vi "UI_Set_startup_controls_state_(01).vi"(3 "error in (no error)":errorcluster, 4 "Settings cluster in":T1={"Defaults"={"Default User"=0.0, "VISA Resource Name "=""}, "Recording and saving"={"Researcher name"="", "Name prefix"="", "Data filtering"=0, "Stop at"=0.0, "\"Stop at\" enabled"=FALSE}, "Geometry"={"Cage diameter, mm"=0, "Starting angle MIDFIELD"=0, "Starting angle BORDER"=0, "Radius, mm CENTER"=0, "Radius, mm MIDFIELD"=0, "N segments MIDFIELD"=0, "N segments BORDER"=0, "R-gap, mm"=0.0, "Bridge swap"=FALSE, "Bridge H. offset"=0.0, "Bridge V. offset"=0.0, "Twisted neck"=FALSE}, "IO parameters"={"SYNC configuration"=0, "IO 1 configuration"=0, "IO 2 configuration"=0, "IO 3 configuration"=0, "IO 4 configuration"=0, "Activate ext. RS-232"=0, "IO inversion config."=0}, "Stimulus presets array"=[{"Event type"=0, "Dur., s"=0.0, "Stim., s"=0.0, "TTL out N"=1, "Set/Clear"=FALSE, "Stim. has been set"=FALSE}, {"Event type"=0, "Dur., s"=0.0, "Stim., s"=0.0, "TTL out N"=1, "Set/Clear"=FALSE, "Stim. has been set"=FALSE}, {"Event type"=0, "Dur., s"=0.0, "Stim., s"=0.0, "TTL out N"=1, "Set/Clear"=FALSE, "Stim. has been set"=FALSE}, {"Event type"=0, "Dur., s"=0.0, "Stim., s"=0.0, "TTL out N"=1, "Set/Clear"=FALSE, "Stim. has been set"=FALSE}, {"Event type"=0, "Dur., s"=0.0, "Stim., s"=0.0, "TTL out N"=1, "Set/Clear"=FALSE, "Stim. has been set"=FALSE}, {"Event type"=0, "Dur., s"=0.0, "Stim., s"=0.0, "TTL out N"=1, "Set/Clear"=FALSE, "Stim. has been set"=FALSE}, {"Event type"=0, "Dur., s"=0.0, "Stim., s"=0.0, "TTL out N"=1, "Set/Clear"=FALSE, "Stim. has been set"=FALSE}, {"Event type"=0, "Dur., s"=0.0, "Stim., s"=0.0, "TTL out N"=1, "Set/Clear"=FALSE, "Stim. has been set"=FALSE}, {"Event type"=0, "Dur., s"=0.0, "Stim., s"=0.0, "TTL out N"=1, "Set/Clear"=FALSE, "Stim. has been set"=FALSE}, {"Event type"=0, "Dur., s"=0.0, "Stim., s"=0.0, "TTL out N"=1, "Set/Clear"=FALSE, "Stim. has been set"=FALSE}, {"Event type"=0, "Dur., s"=0.0, "Stim., s"=0.0, "TTL out N"=1, "Set/Clear"=FALSE, "Stim. has been set"=FALSE}, {"Event type"=0, "Dur., s"=0.0, "Stim., s"=0.0, "TTL out N"=1, "Set/Clear"=FALSE, "Stim. has been set"=FALSE}, {"Event type"=0, "Dur., s"=0.0, "Stim., s"=0.0, "TTL out N"=1, "Set/Clear"=FALSE, "Stim. has been set"=FALSE}, {"Event type"=0, "Dur., s"=0.0, "Stim., s"=0.0, "TTL out N"=1, "Set/Clear"=FALSE, "Stim. has been set"=FALSE}], "Settings loaded OK"=FALSE} {"Stimulus presets array"."Event type" items=["Stay for N seconds"]; "Stimulus presets array"."TTL out N" items=["1"=1, "2"=2, "1+2"=3]; "Geometry"."Cage diameter, mm" scale=0.0..340.0}, 5 "All references in":T5) -> (0 "error out":errorcluster, 1 "Settings cluster out":T1={"Defaults"={"Default User"=0.0, "VISA Resource Name "=""}, "Recording and saving"={"Researcher name"="", "Name prefix"="", "Data filtering"=0, "Stop at"=0.0, "\"Stop at\" enabled"=FALSE}, "Geometry"={"Cage diameter, mm"=0, "Starting angle MIDFIELD"=0, "Starting angle BORDER"=0, "Radius, mm CENTER"=0, "Radius, mm MIDFIELD"=0, "N segments MIDFIELD"=0, "N segments BORDER"=0, "R-gap, mm"=0.0, "Bridge swap"=FALSE, "Bridge H. offset"=0.0, "Bridge V. offset"=0.0, "Twisted neck"=FALSE}, "IO parameters"={"SYNC configuration"=0, "IO 1 configuration"=0, "IO 2 configuration"=0, "IO 3 configuration"=0, "IO 4 configuration"=0, "Activate ext. RS-232"=0, "IO inversion config."=0}, "Stimulus presets array"=[{"Event type"=0, "Dur., s"=0.0, "Stim., s"=0.0, "TTL out N"=1, "Set/Clear"=FALSE, "Stim. has been set"=FALSE}, {"Event type"=0, "Dur., s"=0.0, "Stim., s"=0.0, "TTL out N"=1, "Set/Clear"=FALSE, "Stim. has been set"=FALSE}, {"Event type"=0, "Dur., s"=0.0, "Stim., s"=0.0, "TTL out N"=1, "Set/Clear"=FALSE, "Stim. has been set"=FALSE}, {"Event type"=0, "Dur., s"=0.0, "Stim., s"=0.0, "TTL out N"=1, "Set/Clear"=FALSE, "Stim. has been set"=FALSE}, {"Event type"=0, "Dur., s"=0.0, "Stim., s"=0.0, "TTL out N"=1, "Set/Clear"=FALSE, "Stim. has been set"=FALSE}, {"Event type"=0, "Dur., s"=0.0, "Stim., s"=0.0, "TTL out N"=1, "Set/Clear"=FALSE, "Stim. has been set"=FALSE}, {"Event type"=0, "Dur., s"=0.0, "Stim., s"=0.0, "TTL out N"=1, "Set/Clear"=FALSE, "Stim. has been set"=FALSE}, {"Event type"=0, "Dur., s"=0.0, "Stim., s"=0.0, "TTL out N"=1, "Set/Clear"=FALSE, "Stim. has been set"=FALSE}, {"Event type"=0, "Dur., s"=0.0, "Stim., s"=0.0, "TTL out N"=1, "Set/Clear"=FALSE, "Stim. has been set"=FALSE}, {"Event type"=0, "Dur., s"=0.0, "Stim., s"=0.0, "TTL out N"=1, "Set/Clear"=FALSE, "Stim. has been set"=FALSE}, {"Event type"=0, "Dur., s"=0.0, "Stim., s"=0.0, "TTL out N"=1, "Set/Clear"=FALSE, "Stim. has been set"=FALSE}, {"Event type"=0, "Dur., s"=0.0, "Stim., s"=0.0, "TTL out N"=1, "Set/Clear"=FALSE, "Stim. has been set"=FALSE}, {"Event type"=0, "Dur., s"=0.0, "Stim., s"=0.0, "TTL out N"=1, "Set/Clear"=FALSE, "Stim. has been set"=FALSE}, {"Event type"=0, "Dur., s"=0.0, "Stim., s"=0.0, "TTL out N"=1, "Set/Clear"=FALSE, "Stim. has been set"=FALSE}], "Settings loaded OK"=FALSE} {"Stimulus presets array"."Event type" items=["Stay for N seconds"]; "Stimulus presets array"."TTL out N" items=["1"=1, "2"=2, "1+2"=3]; "Geometry"."Cage diameter, mm" scale=0.0..340.0}, 2 "All references out":T5)   [LabVIEW 2018]
uses:
  Controls/CTL_All_References.ctl
  Controls/CTL_Controls_References.ctl
  Controls/CTL_Indicators_References.ctl
  Controls/CTL_Panes_and_VIs_References.ctl
  Controls/CTL_Histogram_Properties.ctl
  <vilib>/Utility/miscctls.llb/LVRangeTypeDef.ctl
  Controls/CTL_Settings_cluster.ctl
  Controls/CTL_Single_stimulus_setting.ctl
  <vilib>/Utility/error.llb/Error Cluster From Error Code.vi
  <vilib>/ErrorRing/Error Ring.xnode
panel:
  out "Erroneous ref name":string
  in  "Histogram initialization cluster":T3={"X Scale.Range"={"Minimum"=0.0, "Maximum"=13.0, "Increment"=1.0, "Minor Increment"=1.0, "Start"=0.0}, "Caption.Text"="Zone preference (normalized)", "X Scale.Offset and Multiplier:Multiplier"=1.0, "X Scale.Offset and Multiplier:Offset"=0.0, "X Scale.Scale Fit"=2, "X Scale.Display Format:Precision"=0, "Y Scale.Mapping Mode"=0, "Zones preference empty initialized array"=[0, 0, 0, 0, 0, 0, 0, 0, 0, 0, 0, 0, 0, 0], "Plot.Fill/Point Color"=15790320}
  out "Panes references":T8
  out "Controls references params":string[][](array[string])
  out "Indicators references params":string[][](array[string])
  out "Indicators references":T7
  out "Controls references":T6
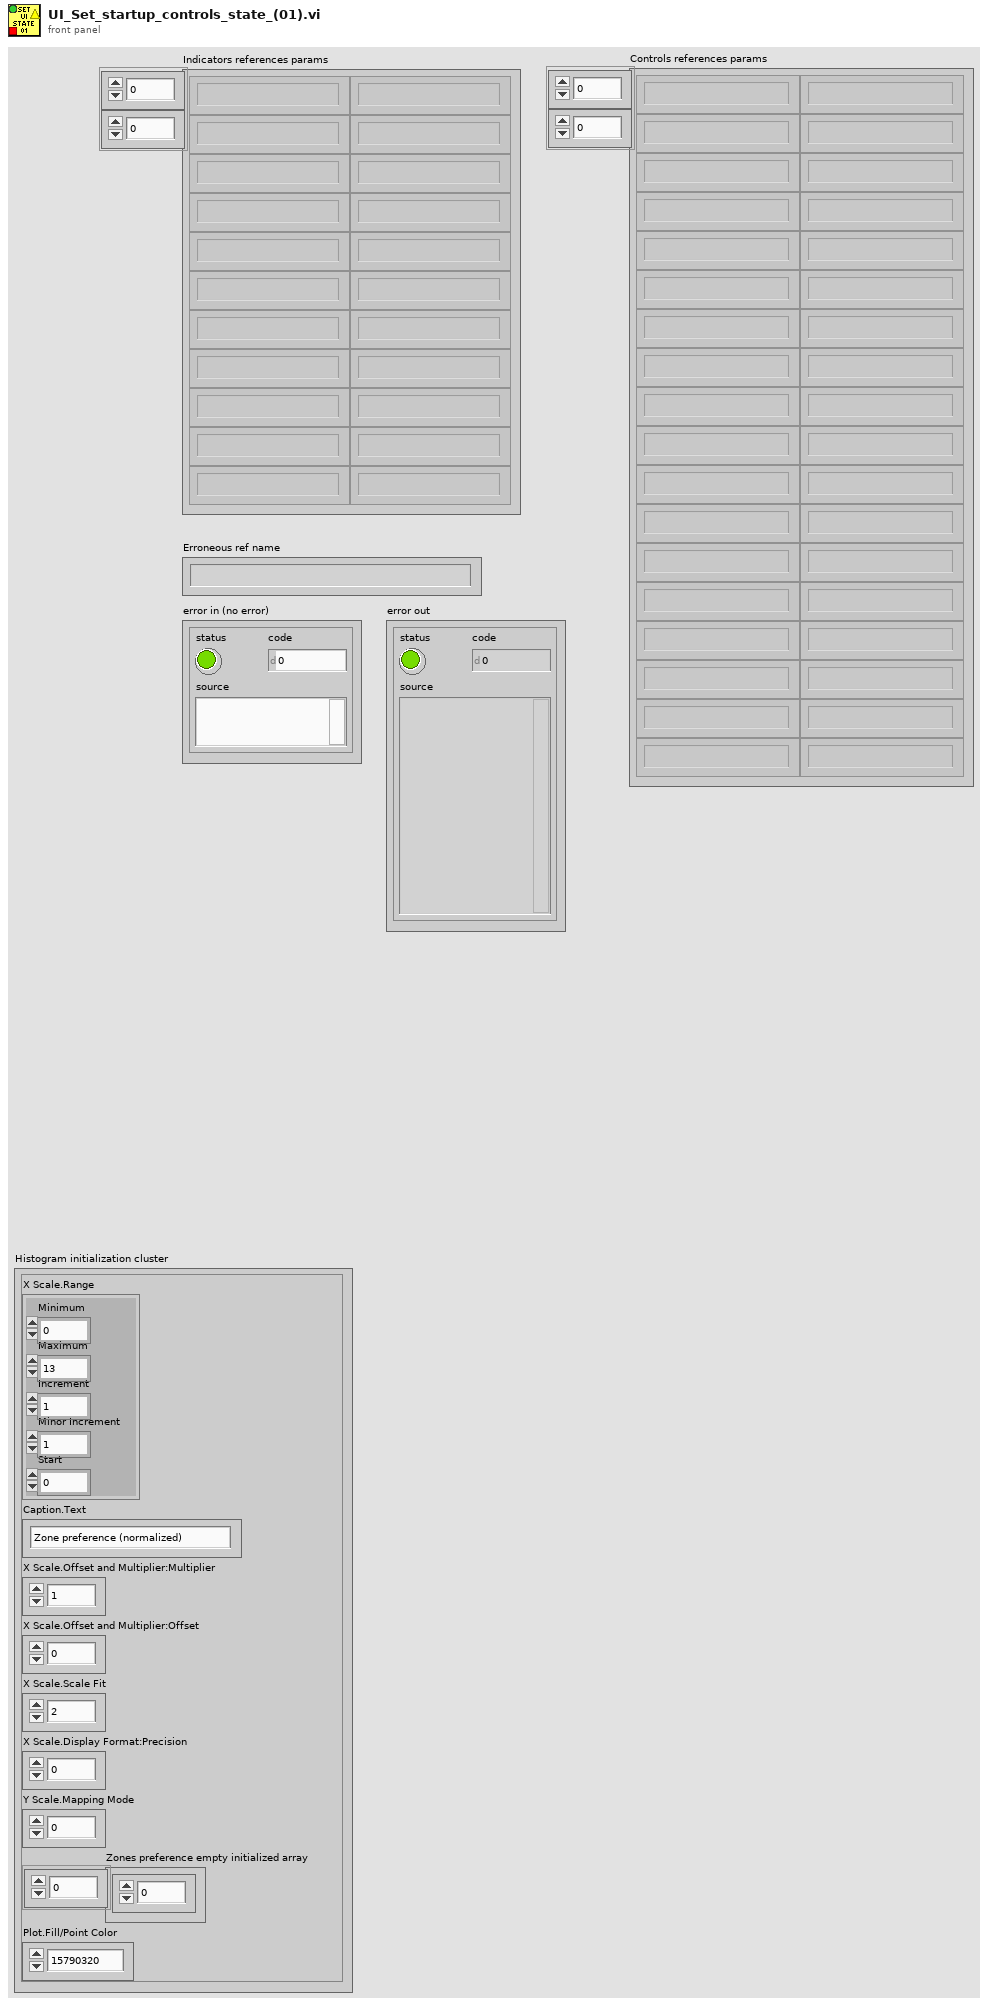
[diagram p1: front panel]
types:
  T1 = typedef "CTL_Settings_cluster.ctl" = cluster{"Defaults":cluster{"Default User":dbl, "VISA Resource Name ":string}, "Recording and saving":cluster{"Researcher name":string, "Name prefix":string, "Data filtering":u16, "Stop at":dbl, "\"Stop at\" enabled":bool}, "Geometry":cluster{"Cage diameter, mm":u16, "Starting angle MIDFIELD":i16, "Starting angle BORDER":i16, "Radius, mm CENTER":u16, "Radius, mm MIDFIELD":u16, "N segments MIDFIELD":u8, "N segments BORDER":u8, "R-gap, mm":sgl, "Bridge swap":bool, "Bridge H. offset":sgl, "Bridge V. offset":sgl, "Twisted neck":bool}, "IO parameters":cluster{"SYNC configuration":u16, "IO 1 configuration":u16, "IO 2 configuration":u16, "IO 3 configuration":u16, "IO 4 configuration":u16, "Activate ext. RS-232":u16, "IO inversion config.":u16}, "Stimulus presets array":T2[], "Settings loaded OK":bool}
  T2 = typedef "CTL_Single_stimulus_setting.ctl" = cluster{"Event type":u16, "Dur., s":sgl, "Stim., s":sgl, "TTL out N":u16, "Set/Clear":bool, "Stim. has been set":bool}
  T3 = typedef "CTL_Histogram_Properties.ctl" = cluster{"X Scale.Range":T4, "Caption.Text":string, "X Scale.Offset and Multiplier:Multiplier":dbl, "X Scale.Offset and Multiplier:Offset":dbl, "X Scale.Scale Fit":u8, "X Scale.Display Format:Precision":u8, "Y Scale.Mapping Mode":u8, "Zones preference empty initialized array":i32[], "Plot.Fill/Point Color":u32}
  T4 = typedef "LVRangeTypeDef.ctl" = cluster{"Minimum":dbl, "Maximum":dbl, "Increment":dbl, "Minor Increment":dbl, "Start":dbl}
  T5 = typedef "CTL_All_References.ctl" = cluster{"Controls references":T6, "Indicators references":T7, "Panes references":T8}
  T6 = typedef "CTL_Controls_References.ctl" = cluster{"Check HW connection":refnum<vi>, "Start Tracking button":refnum<vi>, "Reset zones":refnum<vi>, "Reset stimuli":refnum<vi>, "Record/Stop":refnum<vi>, "Reset barplot":refnum<vi>, "Multiplyer of chart RX":refnum<vi>, "Show zones":refnum<vi>, "Show magnets":refnum<vi>, "Show heatmap":refnum<vi>, "Show full track":refnum<vi>, "Open File":refnum<vi>, "Play/Pause":refnum<vi>, "Trace, s":refnum<vi>, "Playback speed":refnum<vi>, "Timeline":refnum<vi>, "By Zone stim. setup":refnum<vi>}
  T7 = typedef "CTL_Indicators_References.ctl" = cluster{"HW info":refnum<vi>, "Port":refnum<vi>, "Ready":refnum<vi>, "IO status indicator":refnum<vi>, "Current Time":refnum<vi>, "Record timestamp":refnum<vi>, "Mouse speed":refnum<vi>, "Mouse speed, mm/s":refnum<vi>, "Running, perc. of time":refnum<vi>, "Histograms":refnum<vi>}
  T8 = typedef "CTL_Panes_and_VIs_References.ctl" = cluster{"Pane":refnum<vi>, "This VI":refnum<vi>}
  T9 = cluster{"SYNC configuration":u16, "IO 1 configuration":u16, "IO 2 configuration":u16, "IO 3 configuration":u16, "IO 4 configuration":u16, "Activate ext. RS-232":u16, "IO inversion config.":u16}
  T10 = enum8{"Enabled", "Disabled", "Disabled and Grayed Out"}
  T11 = typedef "CTL_IO_parameters_indicator.ctl" = cluster{"IO1":bool, "IO2":bool, "IO3":bool, "IO4":bool, "Z1":bool, "Z2":bool, "Z3":bool, "Z4":bool, "St1":bool, "St2":bool, "St3":bool, "St4":bool, "Syn1":bool, "Syn2":bool, "RS-232 ext. activated":bool}
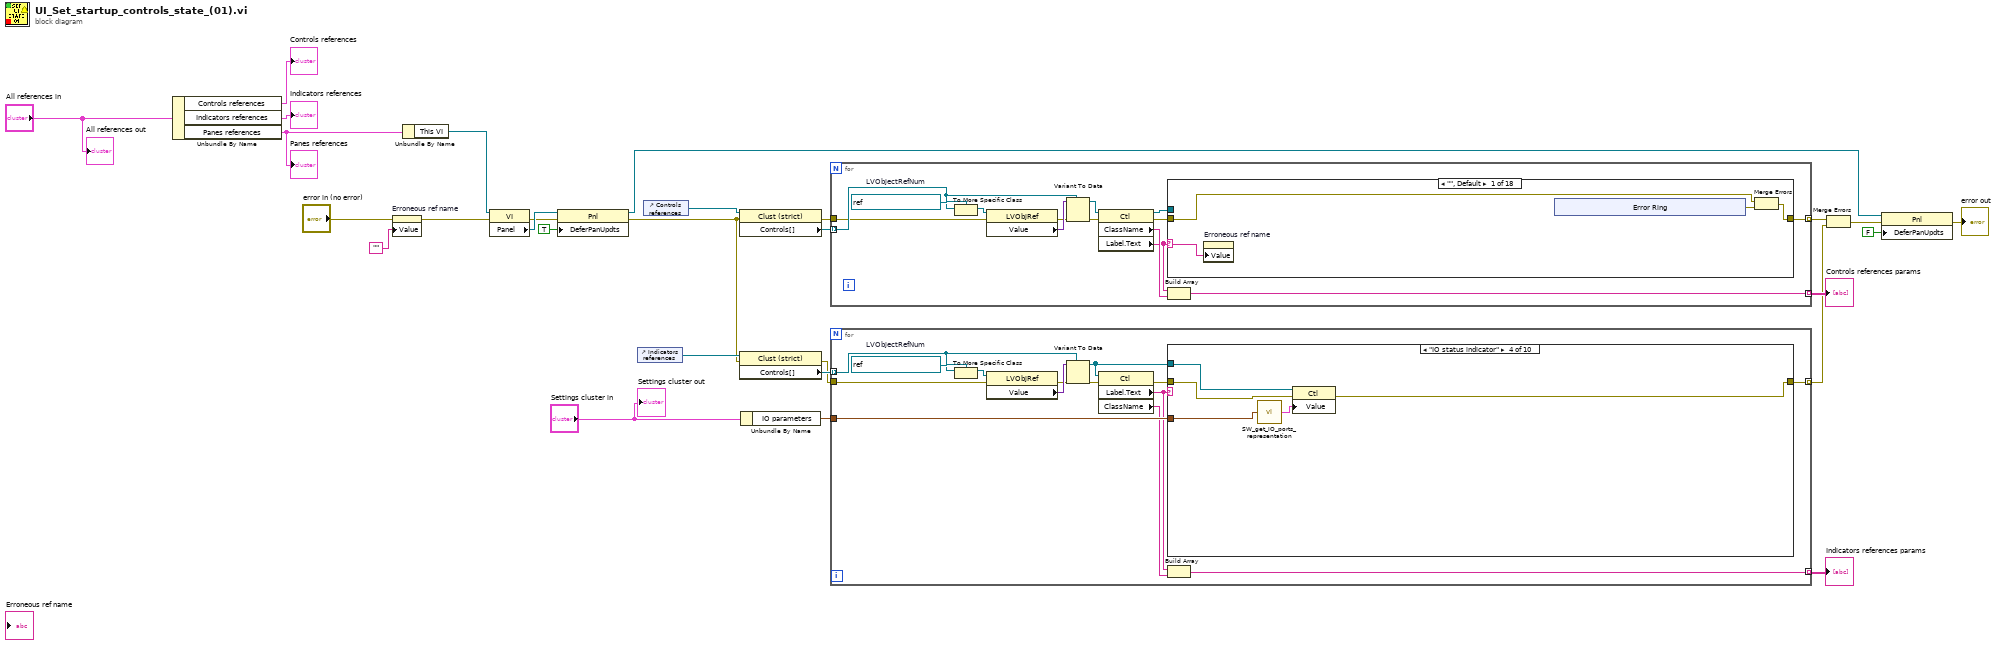
[diagram p0: block diagram]
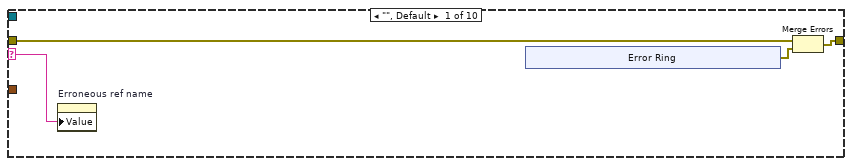
[diagram p2: hidden frame]
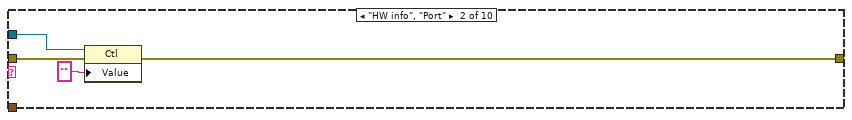
[diagram p3: hidden frame]
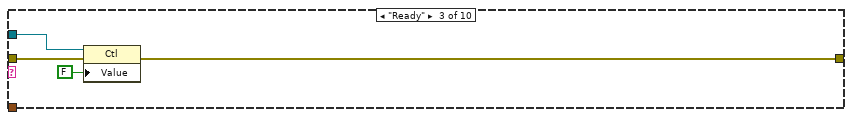
[diagram p4: hidden frame]
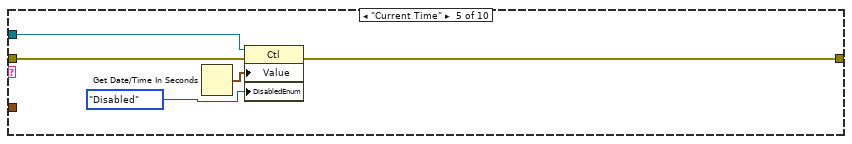
[diagram p5: hidden frame]
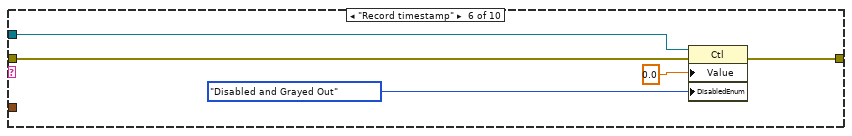
[diagram p6: hidden frame]
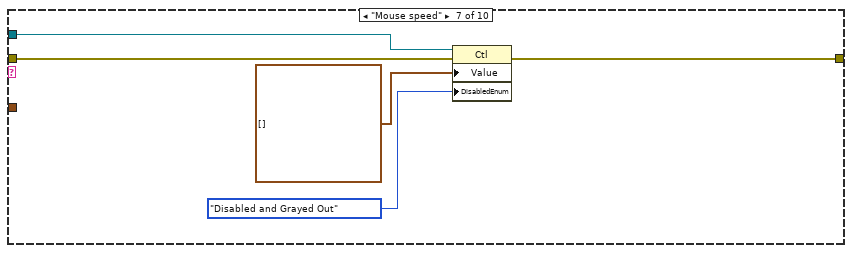
[diagram p7: hidden frame]
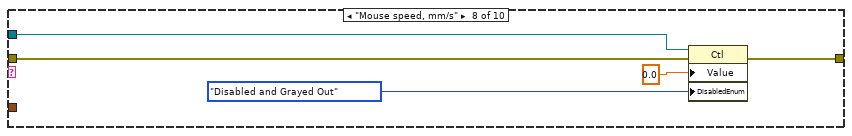
[diagram p8: hidden frame]
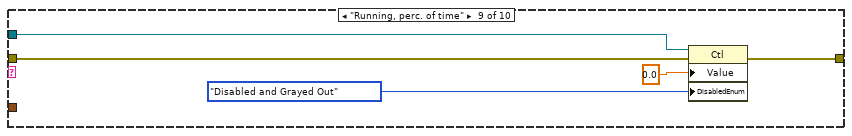
[diagram p9: hidden frame]
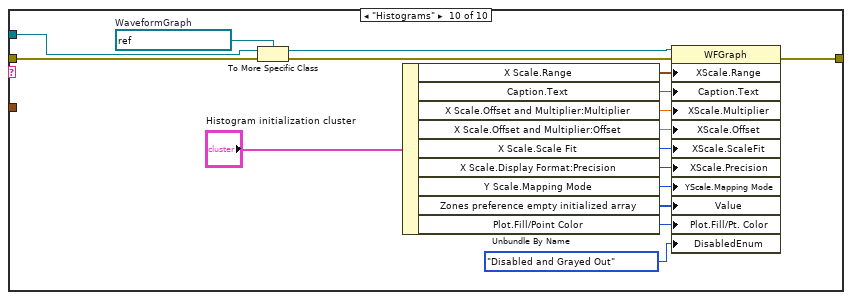
[diagram p10: hidden frame]
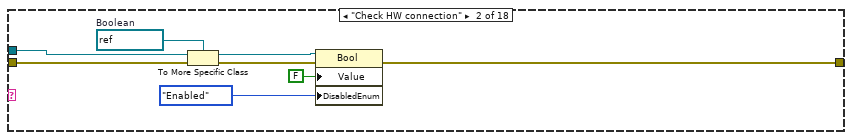
[diagram p11: hidden frame]
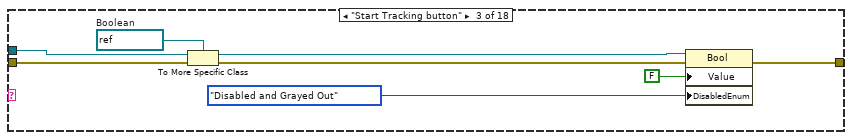
[diagram p12: hidden frame]
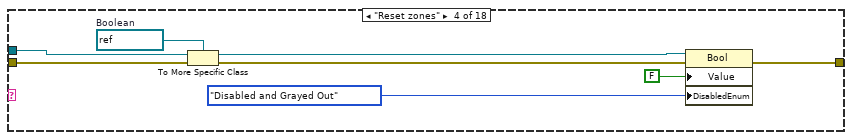
[diagram p13: hidden frame]
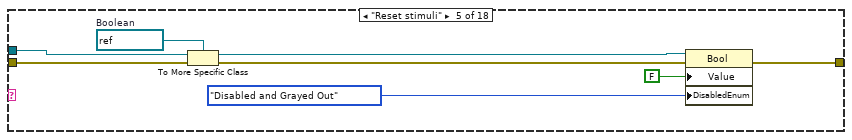
[diagram p14: hidden frame]
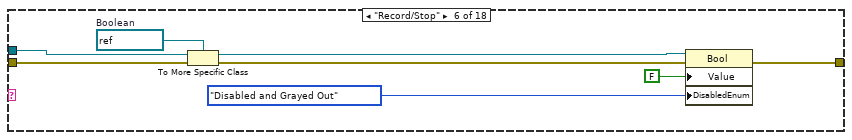
[diagram p15: hidden frame]
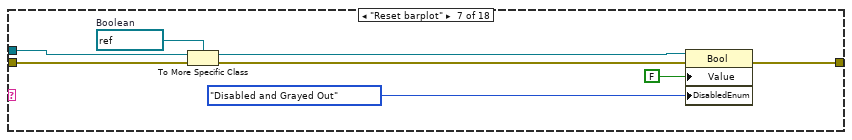
[diagram p16: hidden frame]
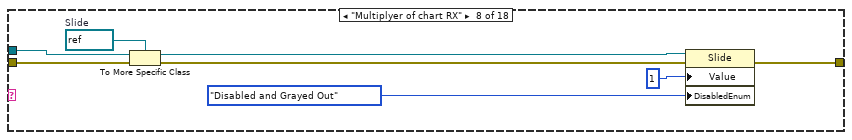
[diagram p17: hidden frame]
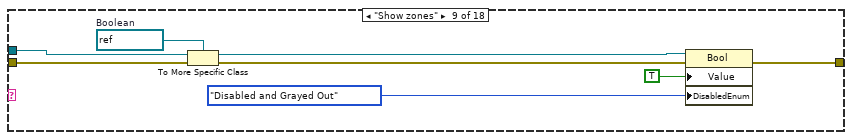
[diagram p18: hidden frame]
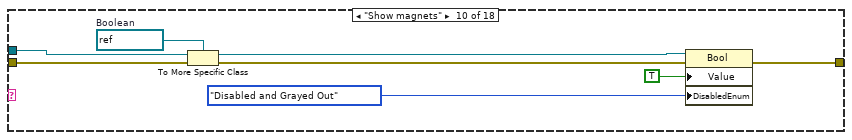
[diagram p19: hidden frame]
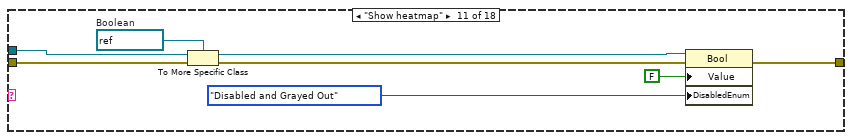
[diagram p20: hidden frame]
diagram:
  n1 = Unbundle By Name("All references in") -> ("Controls references"=→"Controls references":T6, "Indicators references"=→"Indicators references":T7, "Panes references"=w19:T8)
  "Panes references" <- w19
  n2 = property on="Erroneous ref name" class="Str"(error in="error in (no error)", "Value"="") -> (error out=w3:errorcluster)  [unwired: 1 in, 1 out]
  n3 = Unbundle By Name(w19) -> ("This VI"=w16:refnum<vi>)
  n4 = property class="VI"(reference=w16, error in=w3) -> (error out=w8:errorcluster, "Panel"=w18:refnum<vi>)  [unwired: 1 out]
  n5 = property class="Pnl"(reference=w18, error in=w8, "DeferPanUpdts"=TRUE ("Defer Panel Updates")) -> (reference out=w9:refnum<vi>, error out=w15:errorcluster)
  n6 = control-ref of="Indicators references"() -> (w22:refnum<vi>)
  n7 = control-ref of="Controls references"() -> (w24:refnum<vi>)
  n8 = property class="Clust (strict)"(reference=w24, error in=w15) -> (error out=w14:errorcluster, "Controls[]"=w25:refnum<vi>[])  [unwired: 1 out]
  n9 = property class="Clust (strict)"(reference=w22, error in=w15) -> (error out=w13:errorcluster, "Controls[]"=w23:refnum<vi>[])  [unwired: 1 out]
  n10 = Unbundle By Name("Settings cluster in") -> ("IO parameters"=w1:T9)
  n11 = for {
    tunnel: w25 -> [w39] mode=indexing
    tunnel: [w36] -> w20 mode=indexing
    tunnel: w14 -> [w35]
    tunnel: [w31] -> w6 mode=indexing
    w41 = refnum<vi> refnum  # LVObjectRefNum
    n12 = To More Specific Class(target class=w41, reference=w39) -> (specific class reference=w42:refnum<vi>)  [unwired: 1 in, 1 out]
    n13 = property class="LVObjRef"(reference=w42, error in=w35) -> (error out=w34:errorcluster, "Value"=w40:variant)  [unwired: 1 out]
    n14 = Variant To Data(error in=w34, type=w39, Variant=w40) -> (data=w38:refnum<vi>, error out=w33:errorcluster)
    n15 = property class="Ctl"(reference=w38, error in=w33) -> (reference out=w29:refnum<vi>, error out=w30:errorcluster, "ClassName"=w37:string, "Label.Text"=w32:string)
    n16 = case shown="\"\", Default" w32 {
      selector: w32 -> [w43 _ _ _ _ _ _ _ _ _ _ _ _ _ _ _ _ _]
      tunnel: [w45 w54 w62 w70 w78 w86 w94 w102 w110 w118 w126 w134 w142 w150 w158 w166 w174 w181] -> w31
      tunnel: w30 -> [w46 w56 w64 w72 w80 w88 w96 w104 w112 w120 w128 w136 w144 w152 w160 w168 w176 w183]
      tunnel: w29 -> [_ w59 w67 w75 w83 w91 w99 w107 w115 w123 w131 w139 w147 w155 w163 w171 w179 w186]
      frame "", Default {
        n17 = property on="Erroneous ref name" class="Str"("Value"=w43) -> ()  [unwired: 2 in, 2 out]
        n18 = xnode "Error Ring"() -> ("error out"=w44:errorcluster)
        n19 = Merge Errors(w46, w44) -> (w45:errorcluster)
      }
      frame "Check HW connection" {
        w58 = refnum<vi> refnum  # Boolean
        n20 = To More Specific Class(target class=w58, reference=w59, error in=w56) -> (specific class reference=w57:refnum<vi>, error out=w55:errorcluster)
        n21 = property class="Bool"(reference=w57, error in=w55, "Value"=FALSE, "DisabledEnum"=T10."Enabled" ("Disabled")) -> (error out=w54:errorcluster)  [unwired: 1 out]
      }
      frame "Start Tracking button" {
        w66 = refnum<vi> refnum  # Boolean
        n22 = To More Specific Class(target class=w66, reference=w67, error in=w64) -> (specific class reference=w65:refnum<vi>, error out=w63:errorcluster)
        n23 = property class="Bool"(reference=w65, error in=w63, "Value"=FALSE, "DisabledEnum"=T10."Disabled and Grayed Out" ("Disabled")) -> (error out=w62:errorcluster)  [unwired: 1 out]
      }
      frame "Reset zones" {
        w74 = refnum<vi> refnum  # Boolean
        n24 = To More Specific Class(target class=w74, reference=w75, error in=w72) -> (specific class reference=w73:refnum<vi>, error out=w71:errorcluster)
        n25 = property class="Bool"(reference=w73, error in=w71, "Value"=FALSE, "DisabledEnum"=T10."Disabled and Grayed Out" ("Disabled")) -> (error out=w70:errorcluster)  [unwired: 1 out]
      }
      frame "Reset stimuli" {
        w82 = refnum<vi> refnum  # Boolean
        n26 = To More Specific Class(target class=w82, reference=w83, error in=w80) -> (specific class reference=w81:refnum<vi>, error out=w79:errorcluster)
        n27 = property class="Bool"(reference=w81, error in=w79, "Value"=FALSE, "DisabledEnum"=T10."Disabled and Grayed Out" ("Disabled")) -> (error out=w78:errorcluster)  [unwired: 1 out]
      }
      frame "Record/Stop" {
        w90 = refnum<vi> refnum  # Boolean
        n28 = To More Specific Class(target class=w90, reference=w91, error in=w88) -> (specific class reference=w89:refnum<vi>, error out=w87:errorcluster)
        n29 = property class="Bool"(reference=w89, error in=w87, "Value"=FALSE, "DisabledEnum"=T10."Disabled and Grayed Out" ("Disabled")) -> (error out=w86:errorcluster)  [unwired: 1 out]
      }
      frame "Reset barplot" {
        w98 = refnum<vi> refnum  # Boolean
        n30 = To More Specific Class(target class=w98, reference=w99, error in=w96) -> (specific class reference=w97:refnum<vi>, error out=w95:errorcluster)
        n31 = property class="Bool"(reference=w97, error in=w95, "Value"=FALSE, "DisabledEnum"=T10."Disabled and Grayed Out" ("Disabled")) -> (error out=w94:errorcluster)  [unwired: 1 out]
      }
      frame "Multiplyer of chart RX" {
        w106 = refnum<vi> refnum  # Slide
        n32 = To More Specific Class(target class=w106, reference=w107, error in=w104) -> (specific class reference=w105:refnum<vi>, error out=w103:errorcluster)
        n33 = property class="Slide"(reference=w105, error in=w103, "Value"=u8 1, "DisabledEnum"=T10."Disabled and Grayed Out" ("Disabled")) -> (error out=w102:errorcluster)  [unwired: 1 out]
      }
      frame "Show zones" {
        w114 = refnum<vi> refnum  # Boolean
        n34 = To More Specific Class(target class=w114, reference=w115, error in=w112) -> (specific class reference=w113:refnum<vi>, error out=w111:errorcluster)
        n35 = property class="Bool"(reference=w113, error in=w111, "Value"=TRUE, "DisabledEnum"=T10."Disabled and Grayed Out" ("Disabled")) -> (error out=w110:errorcluster)  [unwired: 1 out]
      }
      frame "Show magnets" {
        w122 = refnum<vi> refnum  # Boolean
        n36 = To More Specific Class(target class=w122, reference=w123, error in=w120) -> (specific class reference=w121:refnum<vi>, error out=w119:errorcluster)
        n37 = property class="Bool"(reference=w121, error in=w119, "Value"=TRUE, "DisabledEnum"=T10."Disabled and Grayed Out" ("Disabled")) -> (error out=w118:errorcluster)  [unwired: 1 out]
      }
      frame "Show heatmap" {
        w130 = refnum<vi> refnum  # Boolean
        n38 = To More Specific Class(target class=w130, reference=w131, error in=w128) -> (specific class reference=w129:refnum<vi>, error out=w127:errorcluster)
        n39 = property class="Bool"(reference=w129, error in=w127, "Value"=FALSE, "DisabledEnum"=T10."Disabled and Grayed Out" ("Disabled")) -> (error out=w126:errorcluster)  [unwired: 1 out]
      }
      frame "Show full track" {
        w138 = refnum<vi> refnum  # Boolean
        n40 = To More Specific Class(target class=w138, reference=w139, error in=w136) -> (specific class reference=w137:refnum<vi>, error out=w135:errorcluster)
        n41 = property class="Bool"(reference=w137, error in=w135, "Value"=FALSE, "DisabledEnum"=T10."Disabled and Grayed Out" ("Disabled")) -> (error out=w134:errorcluster)  [unwired: 1 out]
      }
      frame "Open File" {
        w146 = refnum<vi> refnum  # Boolean
        n42 = To More Specific Class(target class=w146, reference=w147, error in=w144) -> (specific class reference=w145:refnum<vi>, error out=w143:errorcluster)
        n43 = property class="Bool"(reference=w145, error in=w143, "Value"=FALSE, "DisabledEnum"=T10."Disabled and Grayed Out" ("Disabled")) -> (error out=w142:errorcluster)  [unwired: 1 out]
      }
      frame "Play/Pause" {
        w154 = refnum<vi> refnum  # Boolean
        n44 = To More Specific Class(target class=w154, reference=w155, error in=w152) -> (specific class reference=w153:refnum<vi>, error out=w151:errorcluster)
        n45 = property class="Bool"(reference=w153, error in=w151, "Value"=FALSE, "DisabledEnum"=T10."Disabled and Grayed Out" ("Disabled")) -> (error out=w150:errorcluster)  [unwired: 1 out]
      }
      frame "Trace, s" {
        w162 = refnum<vi> refnum  # Slide
        n46 = To More Specific Class(target class=w162, reference=w163, error in=w160) -> (specific class reference=w161:refnum<vi>, error out=w159:errorcluster)
        n47 = property class="Slide"(reference=w161, error in=w159, "Value"=u8 5, "DisabledEnum"=T10."Disabled and Grayed Out" ("Disabled")) -> (error out=w158:errorcluster)  [unwired: 1 out]
      }
      frame "Playback speed" {
        w170 = refnum<vi> refnum  # Ring
        n48 = To More Specific Class(target class=w170, reference=w171, error in=w168) -> (specific class reference=w169:refnum<vi>, error out=w167:errorcluster)
        n49 = property class="Ring"(reference=w169, error in=w167, "Value"=u8 3, "DisabledEnum"=T10."Disabled and Grayed Out" ("Disabled")) -> (error out=w166:errorcluster)  [unwired: 1 out]
      }
      frame "Timeline" {
        w178 = refnum<vi> refnum  # Slide
        n50 = To More Specific Class(target class=w178, reference=w179, error in=w176) -> (specific class reference=w177:refnum<vi>, error out=w175:errorcluster)
        n51 = property class="Slide"(reference=w177, error in=w175, "Value"=u8 5, "DisabledEnum"=T10."Disabled and Grayed Out" ("Disabled")) -> (error out=w174:errorcluster)  [unwired: 1 out]
      }
      frame "By Zone stim. setup" {
        w185 = refnum<vi> refnum  # RadioButtonsControl
        n52 = To More Specific Class(target class=w185, reference=w186, error in=w183) -> (specific class reference=w184:refnum<vi>, error out=w182:errorcluster)
        n53 = property class="RadioBtnsControl"(reference=w184, error in=w182, "DisabledEnum"=T10."Disabled and Grayed Out" ("Disabled")) -> (error out=w181:errorcluster)  [unwired: 1 out]
      }
    }
    n54 = Build Array(w32, w37) -> (w36:string[])
  }
  "Controls references params" <- w20
  n55 = for {
    tunnel: w23 -> [w197] mode=indexing
    tunnel: [w187] -> w21 mode=indexing
    tunnel: w13 -> [w195]
    tunnel: [w191] -> w12 mode=indexing
    tunnel: w1 -> [w190]
    w199 = refnum<vi> refnum  # LVObjectRefNum
    n56 = To More Specific Class(target class=w199, reference=w197) -> (specific class reference=w200:refnum<vi>)  [unwired: 1 in, 1 out]
    n57 = property class="LVObjRef"(reference=w200, error in=w195) -> (error out=w194:errorcluster, "Value"=w198:variant)  [unwired: 1 out]
    n58 = Variant To Data(error in=w194, type=w197, Variant=w198) -> (data=w196:refnum<vi>, error out=w193:errorcluster)
    n59 = property class="Ctl"(reference=w196, error in=w193) -> (error out=w192:errorcluster, "Label.Text"=w189:string, "ClassName"=w188:string)  [unwired: 1 out]
    n60 = case shown="\"IO status indicator\"" w189 {
      selector: w189 -> [w204 _ _ _ _ _ _ _ _ _]
      tunnel: w196 -> [_ w213 w217 w219 w227 w232 w237 w242 w247 w264]
      tunnel: w192 -> [w202 w211 w216 w220 w226 w231 w236 w241 w246 w250]
      tunnel: [w201 w210 w215 w222 w225 w230 w235 w240 w245 w263] -> w191
      tunnel: w190 -> [_ _ _ w221 _ _ _ _ _ _]
      frame "", Default {
        n61 = property on="Erroneous ref name" class="Str"("Value"=w204) -> ()  [unwired: 2 in, 2 out]
        n62 = xnode "Error Ring"() -> ("error out"=w203:errorcluster)
        n63 = Merge Errors(w202, w203) -> (w201:errorcluster)
      }
      frame "HW info", "Port" {
        n64 = property class="Ctl"(reference=w213, error in=w211, "Value"="") -> (error out=w210:errorcluster)  [unwired: 1 out]
      }
      frame "Ready" {
        n65 = property class="Ctl"(reference=w217, error in=w216, "Value"=FALSE) -> (error out=w215:errorcluster)  [unwired: 1 out]
      }
      frame "IO status indicator" {
        n66 = call "SW_get_IO_ports_representation.vi"("Sync parameters cluster input"=w221) -> ("IO status indicator"=w218:T11)
        n67 = property class="Ctl"(reference=w219, error in=w220, "Value"=w218) -> (error out=w222:errorcluster)  [unwired: 1 out]
      }
      frame "Current Time" {
        n68 = Get Date/Time In Seconds() -> (seconds since 1Jan1904=w224:timestamp)
        n69 = property class="Ctl"(reference=w227, error in=w226, "Value"=w224, "DisabledEnum"=T10."Disabled" ("Disabled")) -> (error out=w225:errorcluster)  [unwired: 1 out]
      }
      frame "Record timestamp" {
        n70 = property class="Ctl"(reference=w232, error in=w231, "Value"=0.0, "DisabledEnum"=T10."Disabled and Grayed Out" ("Disabled")) -> (error out=w230:errorcluster)  [unwired: 1 out]
      }
      frame "Mouse speed" {
        n71 = property class="Ctl"(reference=w237, error in=w236, "Value"=waveform(dbl)[] [] ("History Data"), "DisabledEnum"=T10."Disabled and Grayed Out" ("Disabled")) -> (error out=w235:errorcluster)  [unwired: 1 out]
      }
      frame "Mouse speed, mm/s" {
        n72 = property class="Ctl"(reference=w242, error in=w241, "Value"=0.0, "DisabledEnum"=T10."Disabled and Grayed Out" ("Disabled")) -> (error out=w240:errorcluster)  [unwired: 1 out]
      }
      frame "Running, perc. of time" {
        n73 = property class="Ctl"(reference=w247, error in=w246, "Value"=0.0, "DisabledEnum"=T10."Disabled and Grayed Out" ("Disabled")) -> (error out=w245:errorcluster)  [unwired: 1 out]
      }
      frame "Histograms" {
        w261 = refnum<vi> refnum  # WaveformGraph
        n74 = To More Specific Class(target class=w261, reference=w264, error in=w250) -> (specific class reference=w262:refnum<vi>, error out=w249:errorcluster)
        n75 = Unbundle By Name("Histogram initialization cluster") -> ("X Scale.Range"=w259:T4, "Caption.Text"=w258:string, "X Scale.Offset and Multiplier:Multiplier"=w257:dbl, "X Scale.Offset and Multiplier:Offset"=w256:dbl, "X Scale.Scale Fit"=w255:u8, "X Scale.Display Format:Precision"=w254:u8, "Y Scale.Mapping Mode"=w253:u8, "Zones preference empty initialized array"=w252:i32[], "Plot.Fill/Point Color"=w251:u32)
        n76 = property class="WFGraph"(reference=w262, error in=w249, "XScale.Range"=w259, "Caption.Text"=w258, "XScale.Multiplier"=w257, "XScale.Offset"=w256, "XScale.ScaleFit"=w255, "XScale.Precision"=w254, "YScale.Mapping Mode"=w253, "Value"=w252, "Plot.Fill/Pt. Color"=w251, "DisabledEnum"=T10."Disabled and Grayed Out" ("Disabled")) -> (error out=w263:errorcluster)  [unwired: 1 out]
      }
    }
    n77 = Build Array(w189, w188) -> (w187:string[])
  }
  "Indicators references params" <- w21
  n78 = Merge Errors(w6, w12) -> (w11:errorcluster)
  n79 = property class="Pnl"(reference=w9, error in=w11, "DeferPanUpdts"=FALSE ("Defer Panel Updates")) -> (error out=→"error out":errorcluster)  [unwired: 1 out]
  "All references out" <- "All references in"
  "Settings cluster out" <- "Settings cluster in"
